vi "Save DUT Information.vi"(8 "error in (no error)":errorcluster, 10 "DUT Info":T1, 11 "TestMonitor in":refnum<class "TestMonitor.lvclass">) -> (0 "error out":errorcluster, 3 "TestMonitor out":refnum<class "TestMonitor.lvclass">)   [LabVIEW 2018, in "TestMonitor.lvclass"]
doc: "This VI will save the DUT Information to the permanent report"
uses:
  TestMonitor.lvclass
  Report Information/DUT Information.ctl
  TestMonitor.lvclass/TestMonitor.ctl
  <vilib>/Skyline/TestMonitor/Test Result/Update Test Result (Single).vi
  <vilib>/Skyline/TestMonitor/Test Result/NI SystemLink Test Result.lvclass
  Report Information/Report Information.lvclass
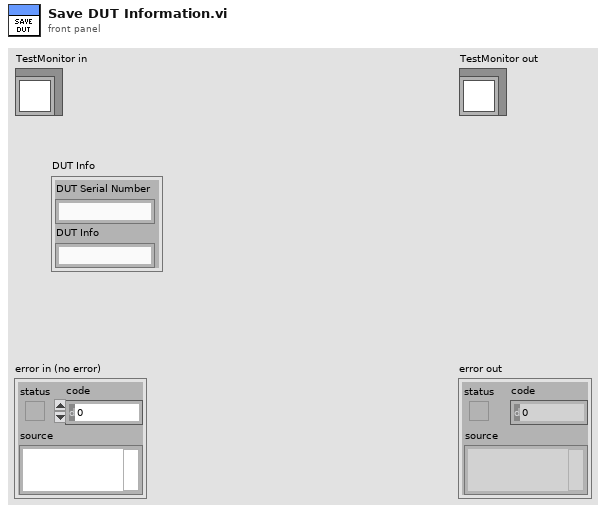
[diagram p1: front panel]
types:
  T1 = typedef "Report Information.lvclass/DUT Information.ctl" = cluster{"DUT Serial Number":string, "DUT Info":string}
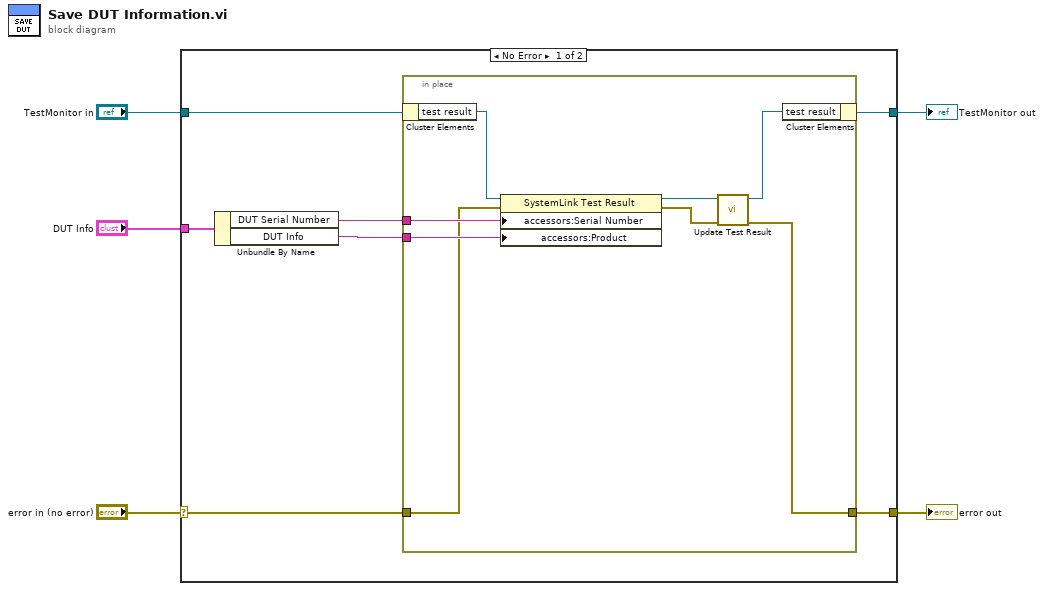
[diagram p0: block diagram]
diagram:
  n1 = case shown="No Error" "error in (no error)" {
    selector: "error in (no error)" -> [w10 w21]
    tunnel: [w11 w21] -> w5
    tunnel: [w9 w22] -> w3
    tunnel: "TestMonitor in" -> [w12 w22]
    tunnel: "DUT Info" -> [w8 _]
    frame No Error {
      n2 = Unbundle By Name(w8) -> ("DUT Serial Number"=w7:string, "DUT Info"=w6:string)
      n3 = in-place {
        in-place-border: [w13] -> w11
        in-place-border: w10 -> [w17]
        in-place-border: w7 -> [w19]
        in-place-border: w6 -> [w18]
        n4 = in-place-cluster #1(w12) -> ("test result"=w20:refnum<class "NI SystemLink Test Result.lvclass">)
        n5 = property class="SystemLink Test Result"(reference=w20, error in=w17, "accessors:Serial Number"=w19, "accessors:Product"=w18) -> (reference out=w16:refnum<class "NI SystemLink Test Result.lvclass">, error out=w14:errorcluster)
        n6 = call-poly <vilib>:"Update Test Result.vi"("error in (no error)"=w14, "test result in"=w16) -> ("error out"=w13:errorcluster, "test result out"=w15:refnum<class "NI SystemLink Test Result.lvclass">)  [unwired: 8 in]
        n7 = in-place-cluster #1("test result"=w15) -> (w9:refnum<class "TestMonitor.lvclass">)
      }
    }
    frame Error {
    }
  }
  "error out" <- w5
  "TestMonitor out" <- w3
